vi "1125_group_6_project.vi"() -> ()   [LabVIEW 2016]
uses:
  <vilib>/DAQmx/write.llb/DAQmx Write (Digital Bool 1Line 1Point).vi
  <vilib>/DAQmx/create/channels.llb/DAQmx Create Channel (DO-Digital Output).vi
  <vilib>/DAQmx/miscellaneous.llb/DAQmx Fill In Error Info.vi
panel:
  in  "Pause":bool
  out "metal_flag":bool
  out "Efficiency":dbl
  out "Total Widgets":dbl
  out "plastic_flag":bool
  out "Widgets Failed":dbl
  out "Widgets Assembled":dbl
  out "Debug Counter":dbl
  out "elements 2":bool[](array[boolean])
  out "Hopper count":dbl
  out "latch for top thing":bool
  out "x > y?":bool
  out "reject/dont":bool
  out "elements":bool[](array[boolean])
  out "latch":bool
  out "laser near rejecter":bool
  out "laser latch":bool
  out "reject_laser":bool
  out "assm_check":bool
  out "bott_laser":bool
  out "bott_ind":bool
  out "bottom sensor":bool
  in  "Reset":bool
  out "ICT_stop":bool
  out "ICT_start":bool
  in  "stop":bool
  out "top_opt":bool
  out "top_ind":bool
  # "Normally On"
  # "Normally On"
  # "Normally On"
  # "Normally On"
  # "For backend data logging, ignore"
  # "Ignore, for debugging"
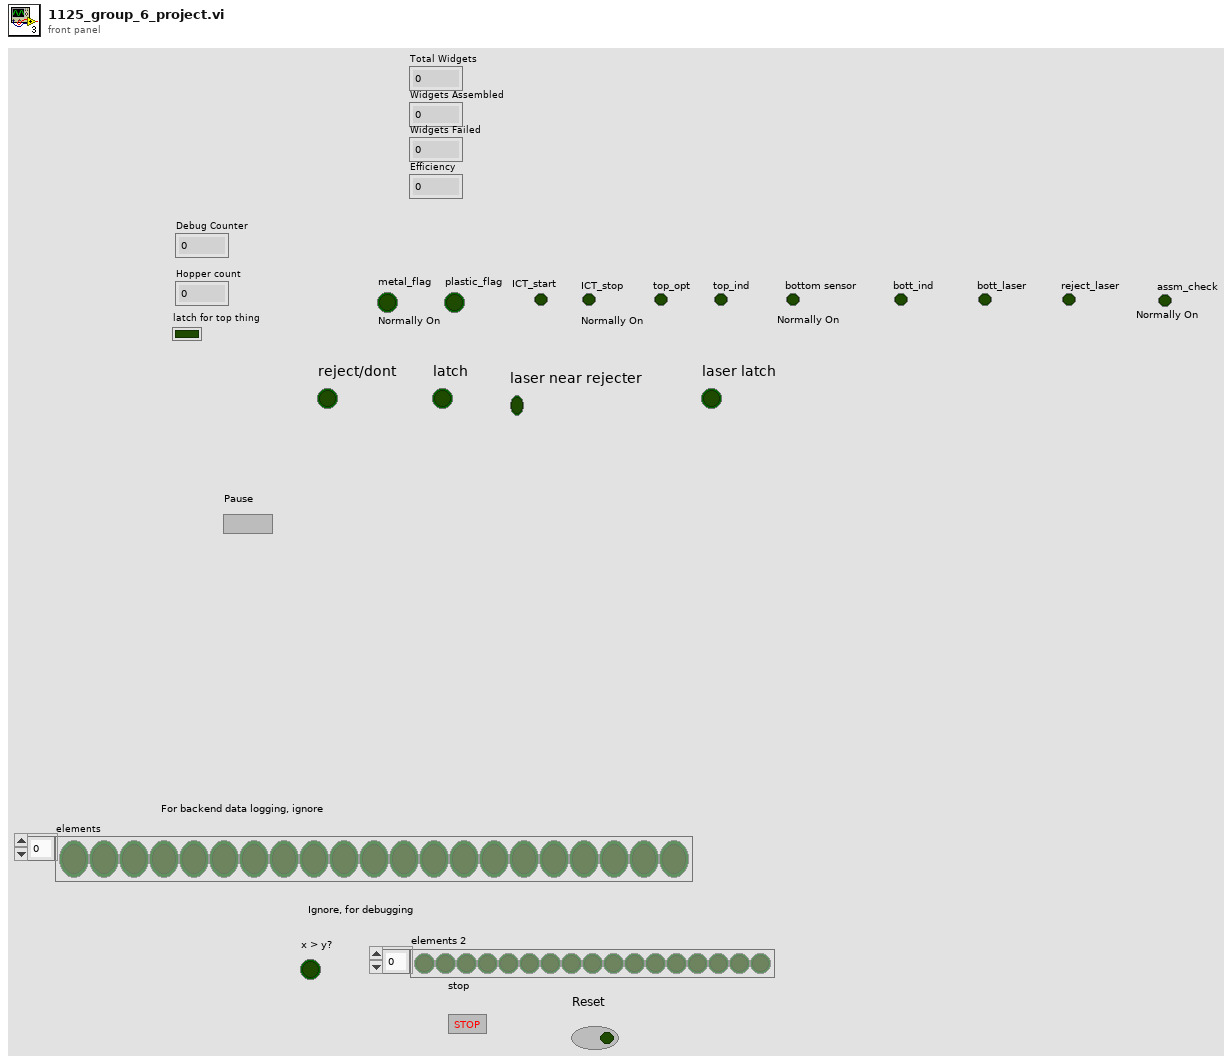
[diagram p1: front panel]
types:
  T1 = enum16{"open", "replace", "create", "open or create", "replace or create", "replace or create with confirmation"}
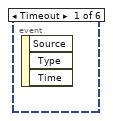
[diagram p4: hidden frame]
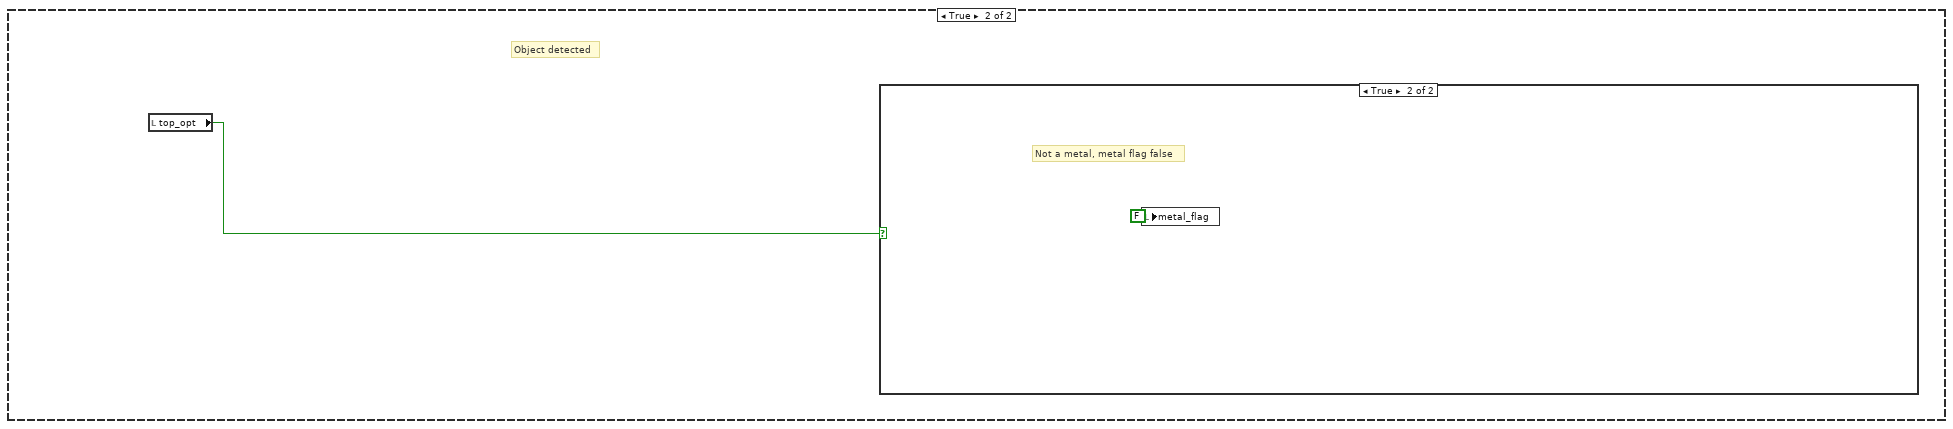
[diagram p8: hidden frame]
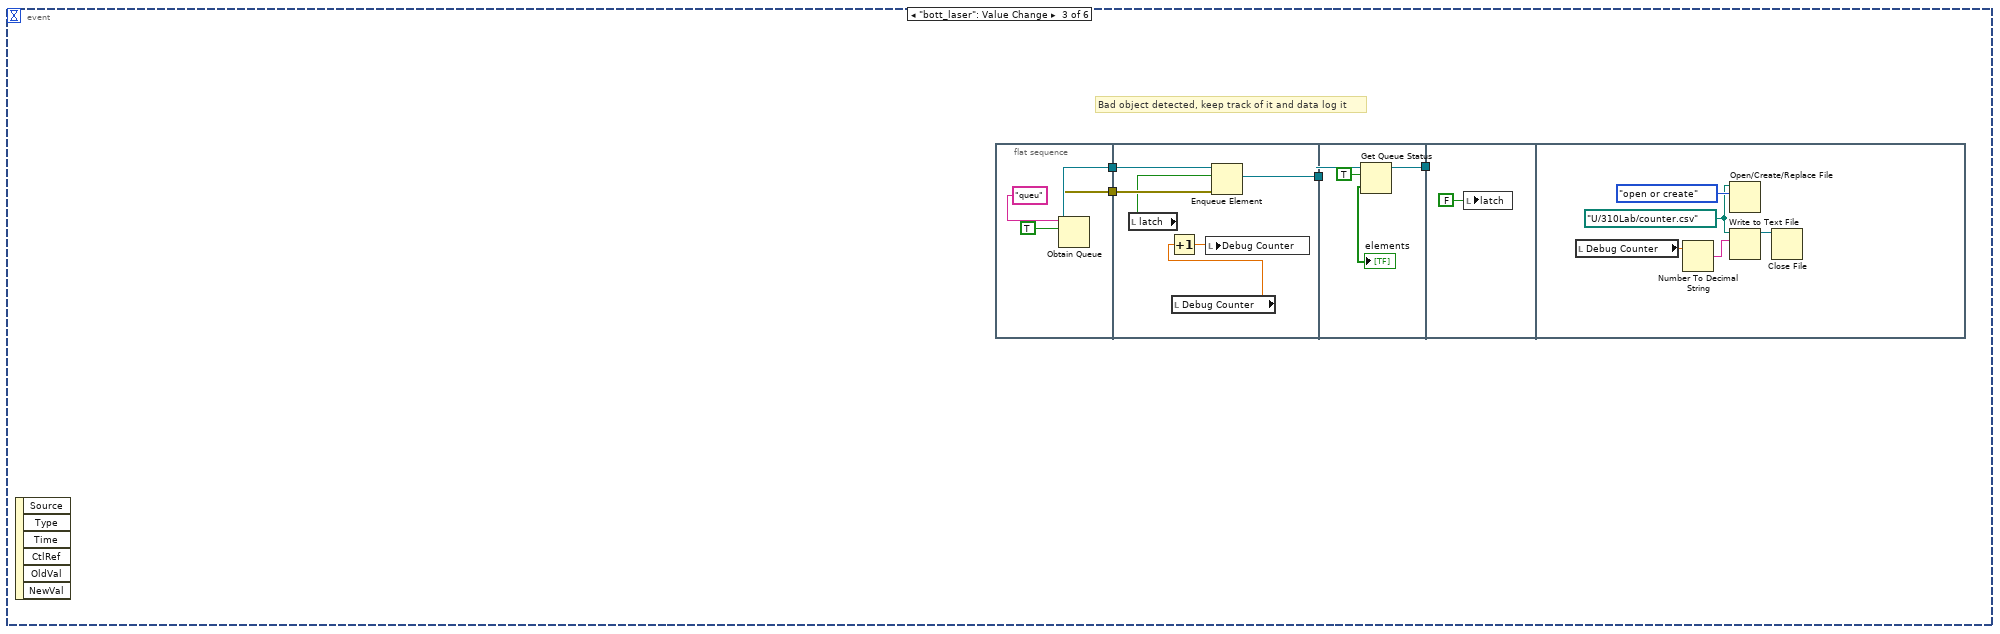
[diagram p10: hidden frame]
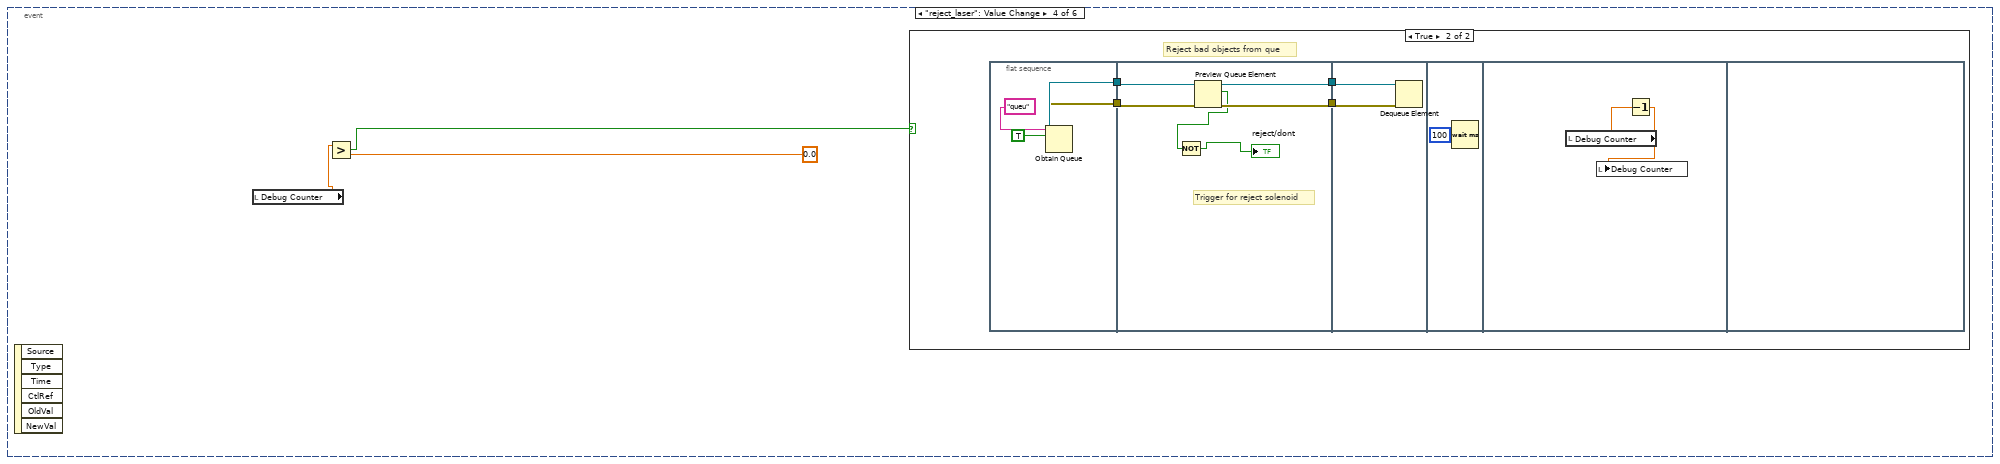
[diagram p11: hidden frame]
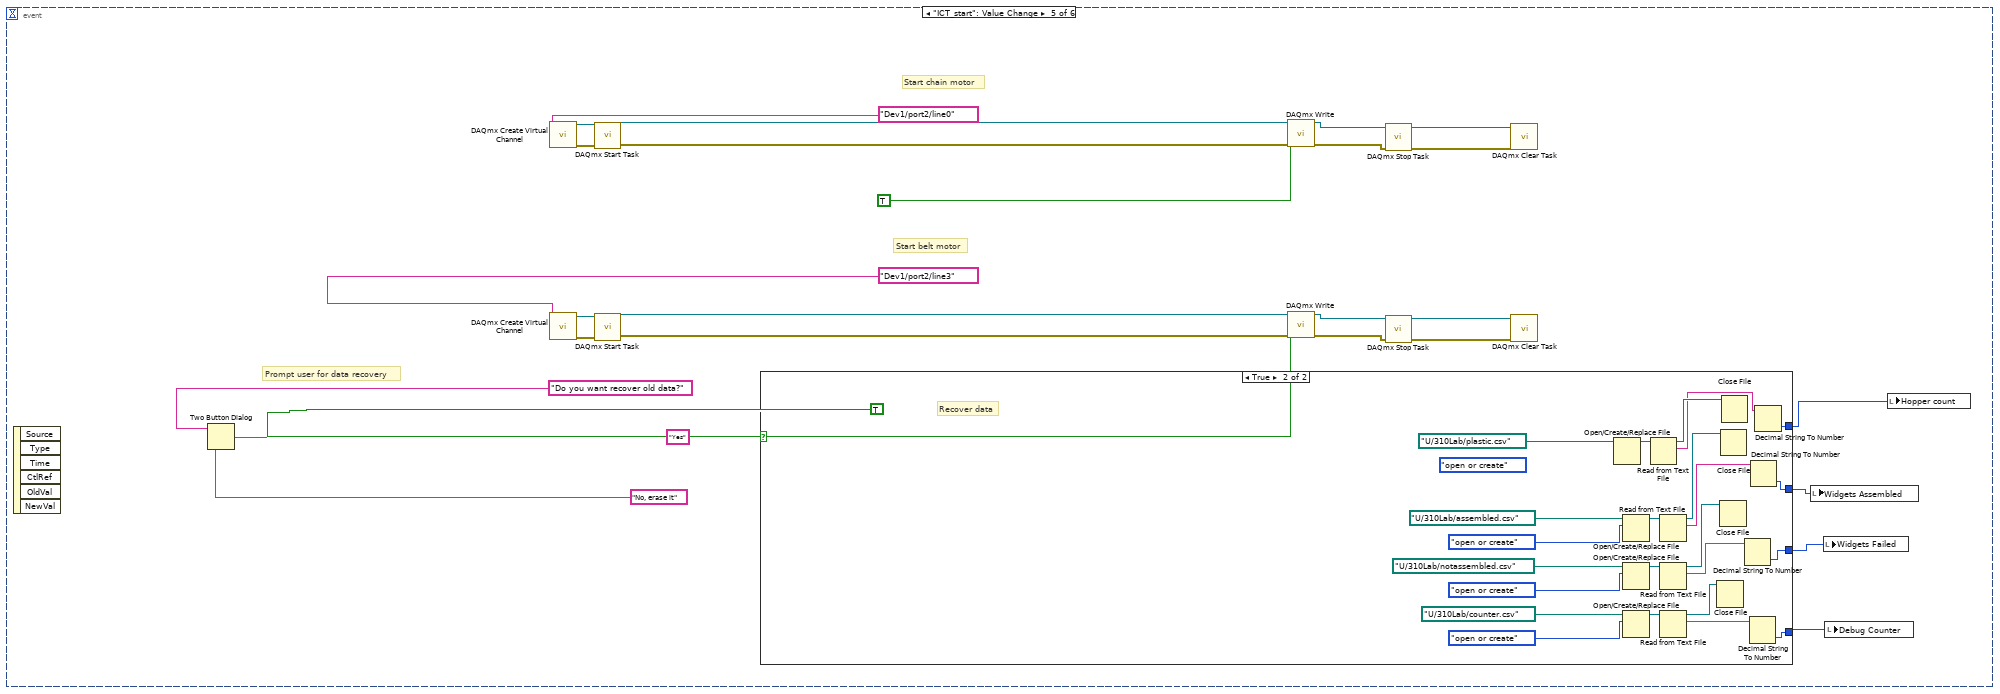
[diagram p13: hidden frame]
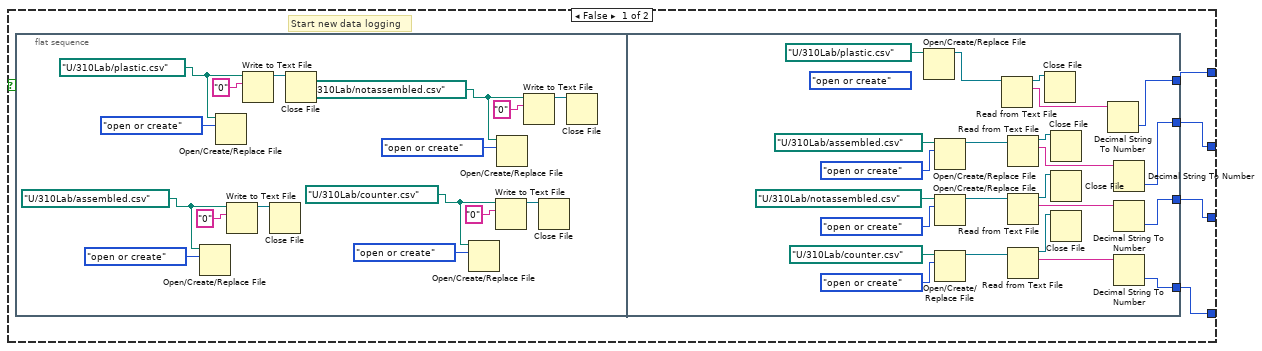
[diagram p14: hidden frame]
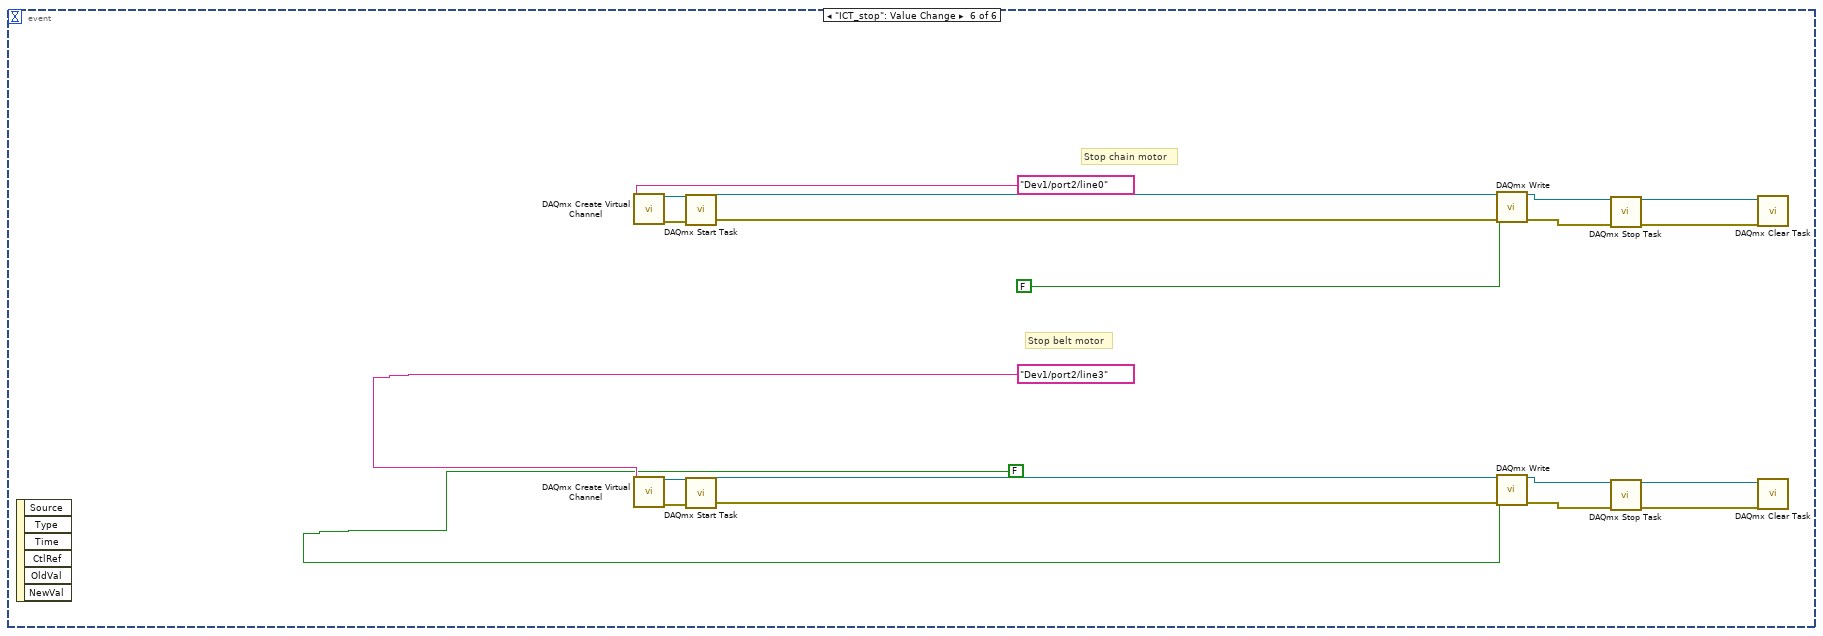
[diagram p15: hidden frame]
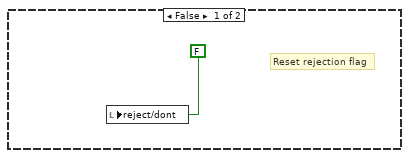
[diagram p19: hidden frame]
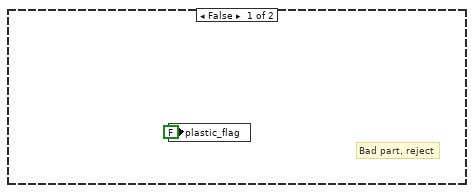
[diagram p20: hidden frame]
diagram:
  n1 = while {
    shift-right: [w60] -> _
    shift-left: _ -> [w61]
    shift-right: [w55] -> _
    shift-left: _ -> [w53]
    shift-right: [w51] -> _
    shift-left: _ -> [w50]
    shift-right: [w46] -> _
    shift-left: _ -> [w45]
    shift-right: [w39] -> _
    shift-left: _ -> [w36]
    shift-right: [w37] -> _
    shift-left: _ -> [w30]
    shift-right: [w38] -> _
    shift-left: _ -> [w28]
    shift-right: [w26] -> _
    shift-left: _ -> [w25]
    shift-right: [w21] -> _
    shift-left: _ -> [w20]
    shift-right: [w13] -> _
    shift-left: _ -> [w12]
    stop <- "stop" stop-if-true
    # "Bottom thing read vi"
    # "Bottom solenoid VI"
    # "Bottom metal sensor VI"
    # "Assembly check read VI"
    # "Dropper read VI"
    # "Stop button VI"
    # "Start button VI"
    # "Final Check"
    # "Shift registers to keep dynamic variables alive"
    # "Variables declaration"
    # "Reset all values stored (debugging purposes)"
    # "Ignore, for Debugging"
    # "Flag that metal is on chain"
    # "Read top_opt sensorr VI"
    # "Read top induct_sensor VI"
    # "Store top_opt status with shift register"
    # "Store top_ind status with shift register"
    # "Efficiency Calculation"
    n2 = local read "Widgets Assembled"() -> (w6:dbl)
    n3 = local read "Widgets Failed"() -> (w9:dbl)
    n4 = flat-sequence {
      frame #0 {
        n5 = event shown="[1] \"top_opt\": Value Change" {
          selector: _ -> [_ _ _ _ _ _]
          dyn-events: _ -> [_ _ _ _ _ _]
          timeout: 10 -> [_ _ _ _ _ _]
          event Timeout {
            n6 = event-data() -> ()  [unwired: 1 in, 3 out]
          }
          event "top_opt": Value Change {
            n7 = event-data() -> ()  [unwired: 1 in, 6 out]
            n8 = local read "top_ind"() -> (w73:bool)
            n9 = case shown="False" w73 {
              frame False {
                # "No object at top"
                n10 = local read "metal_flag"() -> (w74:bool)
                n11 = case shown="True" w74 {
                  frame False {
                  }
                  frame True {
                    # "Metal en route"
                    n12 = local read "top_opt"() -> (w75:bool)
                    n13 = case shown="True" w75 {
                      frame False {
                      }
                      frame True {
                        # "Check hopper"
                        # "Plastic ready"
                        n14 = local read "Hopper count"() -> (w77:dbl)
                        n15 = Less?(x=w77, y=5.0) -> (x < y?=w76:bool)
                        n16 = case shown="True" w76 {
                          frame False {
                          }
                          frame True {
                            # "Hopper not full, trigger sequence to add plastic to hopper"
                            n17 = flat-sequence {
                              frame #0 {
                                # "Stop belt motor"
                                n18 = call "1125_digital_write.vi"("lines"=tag "Dev1/port2/line3", "top ac"=FALSE ("top ac 2")) -> ()  [unwired: 10 in]
                              }
                              frame #1 {
                                # "Stop chain motor"
                                n19 = call "1125_digital_write.vi"("lines"=tag "Dev1/port2/line0", "top ac"=FALSE ("top ac 2")) -> ()  [unwired: 10 in]
                              }
                              frame #2 {
                                # "Enable sort solenoid"
                                n20 = call "1125_digital_write.vi"("lines"=tag "Dev1/port2/line1", "top ac"=TRUE ("top ac 2")) -> ()  [unwired: 10 in]
                              }
                              frame #3 {
                                n21 = Wait (ms)(milliseconds to wait=u32 500) -> ()  [unwired: 1 out]
                              }
                              frame #4 {
                                n22 = Wait (ms)(milliseconds to wait=u32 300) -> ()  [unwired: 1 out]
                              }
                              frame #5 {
                                # "Disable sort solenoid"
                                n23 = call "1125_digital_write.vi"("lines"=tag "Dev1/port2/line1", "top ac"=FALSE ("top ac 2")) -> ()  [unwired: 10 in]
                              }
                              frame #6 {
                                # "Add to hopper count"
                                n24 = local read "Hopper count"() -> (w90:dbl)
                                n25 = Add(x=w90, y=1.0) -> (x+y=w91:dbl)
                                n26 = local write "Hopper count"(w91) -> ()
                              }
                              frame #7 {
                                w95 = path "U:/310Lab/plastic.csv" ("file path (use dialog)")
                                # "Log hopper status"
                                n27 = local read "Hopper count"() -> (w94:dbl)
                                n28 = Number To Decimal String(number=w94) -> (decimal integer string=w93:string)  [unwired: 1 in]
                                n29 = Open/Create/Replace File(file path (use dialog)=w95, operation (0:open)=T1."open or create") -> ()  [unwired: 4 in, 3 out]
                                n30 = Write to Text File(file (use dialog)=w95, text=w93) -> (refnum out=w92:refnum<file>)  [unwired: 2 in, 2 out]
                                n31 = Close File(refnum=w92) -> ()  [unwired: 1 in, 2 out]
                              }
                              frame #8 {
                                # "Start belt motor"
                                n32 = call "1125_digital_write.vi"("lines"=tag "Dev1/port2/line0", "top ac"=TRUE ("top ac 2")) -> ()  [unwired: 10 in]
                              }
                              frame #9 {
                                # "Start chain motor"
                                n33 = call "1125_digital_write.vi"("lines"=tag "Dev1/port2/line3", "top ac"=TRUE ("top ac 2")) -> ()  [unwired: 10 in]
                              }
                            }
                          }
                        }
                      }
                    }
                  }
                }
              }
              frame True {
                # "Object detected"
                n34 = local read "top_opt"() -> (w101:bool)
                n35 = case shown="True" w101 {
                  frame False {
                  }
                  frame True {
                    # "Not a metal, metal flag false"
                    n36 = local write "metal_flag"(FALSE ("flag 2")) -> ()
                  }
                }
              }
            }
          }
          event "bott_laser": Value Change {
            # "Bad object detected, keep track of it and data log it"
            n37 = event-data() -> ()  [unwired: 1 in, 6 out]
            n38 = flat-sequence {
              tunnel: [w108] -> w106
              tunnel: [w107] -> w105
              tunnel: [w113] -> w104
              tunnel: w106 -> [w116]
              tunnel: w105 -> [w115]
              tunnel: w104 -> [w118]
              tunnel: [w117] -> w103
              tunnel: w103 -> [_]
              frame #0 {
                n39 = Obtain Queue(name (unnamed)="queu", element data type=TRUE ("latch bot")) -> (queue out=w108:refnum<queue>, error out=w107:errorcluster)  [unwired: 3 in, 1 out]
              }
              frame #1 {
                n40 = local read "latch"() -> (w114:bool)
                n41 = local read "Debug Counter"() -> (w111:dbl)
                n42 = Increment(x=w111) -> (x+1=w112:dbl)
                n43 = local write "Debug Counter"(w112) -> ()
                n44 = Enqueue Element(queue=w116, element=w114, error in (no error)=w115) -> (queue out=w113:refnum<queue>)  [unwired: 1 in, 2 out]
              }
              frame #2 {
                n45 = Get Queue Status(queue=w118, return elements? (F)=TRUE) -> (queue out=w117:refnum<queue>, elements=→"elements":bool[])  [unwired: 1 in, 6 out]
              }
              frame #3 {
                n46 = local write "latch"(FALSE ("latch bot")) -> ()
              }
              frame #4 {
                w125 = path "U:/310Lab/counter.csv" ("file path (use dialog)")
                n47 = local read "Debug Counter"() -> (w124:dbl)
                n48 = Number To Decimal String(number=w124) -> (decimal integer string=w123:string)  [unwired: 1 in]
                n49 = Open/Create/Replace File(file path (use dialog)=w125, operation (0:open)=T1."open or create") -> ()  [unwired: 4 in, 3 out]
                n50 = Write to Text File(file (use dialog)=w125, text=w123) -> (refnum out=w122:refnum<file>)  [unwired: 2 in, 2 out]
                n51 = Close File(refnum=w122) -> ()  [unwired: 1 in, 2 out]
              }
            }
          }
          event "reject_laser": Value Change {
            n52 = event-data() -> ()  [unwired: 1 in, 6 out]
            n53 = local read "Debug Counter"() -> (w129:dbl)
            n54 = Greater?(x=w129, y=0.0) -> (0:w127:bool)
            n55 = case shown="True" w127 {
              frame False {
                # "No bad objects in que"
              }
              frame True {
                # "Reject bad objects from que"
                n56 = flat-sequence {
                  tunnel: [w135] -> w132
                  tunnel: [w134] -> w133
                  tunnel: w133 -> [w139]
                  tunnel: [w141] -> w130
                  tunnel: w132 -> [w143]
                  tunnel: [w142] -> w131
                  tunnel: w131 -> [w145]
                  tunnel: w130 -> [w144]
                  frame #0 {
                    n57 = Obtain Queue(name (unnamed)="queu", element data type=TRUE ("latch bot")) -> (queue out=w135:refnum<queue>, error out=w134:errorcluster)  [unwired: 3 in, 1 out]
                  }
                  frame #1 {
                    # "Trigger for reject solenoid"
                    n58 = Preview Queue Element(queue=w143, error in (no error)=w139) -> (queue out=w142:refnum<queue>, element=w140:bool, error out=w141:errorcluster)  [unwired: 1 in, 1 out]
                    n59 = Not(x=w140) -> (.not. x?=→"reject/dont":bool)
                  }
                  frame #2 {
                    n60 = Dequeue Element(queue=w145, error in (no error)=w144) -> ()  [unwired: 1 in, 4 out]
                  }
                  frame #3 {
                    n61 = Wait (ms)(milliseconds to wait=u32 100) -> ()  [unwired: 1 out]
                  }
                  frame #4 {
                    n62 = local read "Debug Counter"() -> (w148:dbl)
                    n63 = Decrement(x=w148) -> (x-1=w147:dbl)
                    n64 = local write "Debug Counter"(w147) -> ()
                  }
                  frame #5 {
                  }
                }
              }
            }
          }
          event "ICT_start": Value Change {
            # "Prompt user for data recovery"
            # "Start belt motor"
            # "Start chain motor"
            n65 = event-data() -> ()  [unwired: 1 in, 6 out]
            n66 = Two Button Dialog(message="Do you want recover old data?", 1:"No, erase it" ("F button name (\"Cancel\")"), 2:"Yes" ("T button name (\"OK\")")) -> (T button?=w153:bool)
            n67 = call-poly <vilib>:"DAQmx Create Virtual Channel.vi"("lines"=tag "Dev1/port2/line0") -> ("task out"=w175:refnum<k21>, "error out"=w174:errorcluster)  [unwired: 13 in]
            n68 = call-poly <vilib>:"DAQmx Create Virtual Channel.vi"("lines"=tag "Dev1/port2/line3") -> ("task out"=w160:refnum<k21>, "error out"=w161:errorcluster)  [unwired: 13 in]
            n69 = call <vilib>:"DAQmx Start Task.vi"("task/channels in"=w175, "error in"=w174) -> ("task out"=w171:refnum<k21>, "error out"=w168:errorcluster)  [unwired: 12 in]
            n70 = call <vilib>:"DAQmx Start Task.vi"("task/channels in"=w160, "error in"=w161) -> ("task out"=w164:refnum<k21>, "error out"=w167:errorcluster)  [unwired: 12 in]
            n71 = case shown="True" w153 {
              tunnel: [w180 w230] -> w149
              tunnel: [w178 w229] -> w151
              tunnel: [w179 w228] -> w150
              tunnel: [w177 w220] -> w152
              frame False {
                # "Start new data logging"
                n72 = flat-sequence {
                  tunnel: [w217] -> w180
                  tunnel: [w214] -> w179
                  tunnel: [w211] -> w178
                  tunnel: [w197] -> w177
                  frame #0 {
                    w184 = path "U:/310Lab/notassembled.csv" ("file path (use dialog)")
                    w185 = path "U:/310Lab/counter.csv" ("file path (use dialog)")
                    w192 = path "U:/310Lab/assembled.csv" ("file path (use dialog)")
                    w193 = path "U:/310Lab/plastic.csv" ("file path (use dialog)")
                    n73 = Open/Create/Replace File(file path (use dialog)=w192, operation (0:open)=T1."open or create") -> ()  [unwired: 4 in, 3 out]
                    n74 = Open/Create/Replace File(file path (use dialog)=w193, operation (0:open)=T1."open or create") -> ()  [unwired: 4 in, 3 out]
                    n75 = Write to Text File(file (use dialog)=w192, text="0") -> (refnum out=w190:refnum<file>)  [unwired: 2 in, 2 out]
                    n76 = Write to Text File(file (use dialog)=w193, text="0") -> (refnum out=w195:refnum<file>)  [unwired: 2 in, 2 out]
                    n77 = Close File(refnum=w190) -> ()  [unwired: 1 in, 2 out]
                    n78 = Close File(refnum=w195) -> ()  [unwired: 1 in, 2 out]
                    n79 = Open/Create/Replace File(file path (use dialog)=w185, operation (0:open)=T1."open or create") -> ()  [unwired: 4 in, 3 out]
                    n80 = Write to Text File(file (use dialog)=w185, text="0") -> (refnum out=w187:refnum<file>)  [unwired: 2 in, 2 out]
                    n81 = Open/Create/Replace File(file path (use dialog)=w184, operation (0:open)=T1."open or create") -> ()  [unwired: 4 in, 3 out]
                    n82 = Write to Text File(file (use dialog)=w184, text="0") -> (refnum out=w182:refnum<file>)  [unwired: 2 in, 2 out]
                    n83 = Close File(refnum=w187) -> ()  [unwired: 1 in, 2 out]
                    n84 = Close File(refnum=w182) -> ()  [unwired: 1 in, 2 out]
                  }
                  frame #1 {
                    (unwired) T1."open or create" ("operation (0:open)")
                    n85 = Open/Create/Replace File(file path (use dialog)=path "U:/310Lab/plastic.csv") -> (refnum out=w198:refnum<file>)  [unwired: 5 in, 2 out]
                    n86 = Open/Create/Replace File(file path (use dialog)=path "U:/310Lab/assembled.csv", operation (0:open)=T1."open or create") -> (refnum out=w201:refnum<file>)  [unwired: 4 in, 2 out]
                    n87 = Open/Create/Replace File(file path (use dialog)=path "U:/310Lab/notassembled.csv", operation (0:open)=T1."open or create") -> (refnum out=w202:refnum<file>)  [unwired: 4 in, 2 out]
                    n88 = Open/Create/Replace File(file path (use dialog)=path "U:/310Lab/counter.csv", operation (0:open)=T1."open or create") -> (refnum out=w203:refnum<file>)  [unwired: 4 in, 2 out]
                    n89 = Read from Text File(file (use dialog)=w198) -> (refnum out=w199:refnum<file>, text=w200:string)  [unwired: 3 in, 2 out]
                    n90 = Read from Text File(file (use dialog)=w201) -> (refnum out=w213:refnum<file>, text=w212:string)  [unwired: 3 in, 2 out]
                    n91 = Read from Text File(file (use dialog)=w202) -> (refnum out=w215:refnum<file>, text=w216:string)  [unwired: 3 in, 2 out]
                    n92 = Read from Text File(file (use dialog)=w203) -> (refnum out=w219:refnum<file>, text=w218:string)  [unwired: 3 in, 2 out]
                    n93 = Close File(refnum=w199) -> ()  [unwired: 1 in, 2 out]
                    n94 = Close File(refnum=w213) -> ()  [unwired: 1 in, 2 out]
                    n95 = Close File(refnum=w215) -> ()  [unwired: 1 in, 2 out]
                    n96 = Close File(refnum=w219) -> ()  [unwired: 1 in, 2 out]
                    n97 = Decimal String To Number(string=w200) -> (number=w197:i32)  [unwired: 2 in, 1 out]
                    n98 = Decimal String To Number(string=w212) -> (number=w211:i32)  [unwired: 2 in, 1 out]
                    n99 = Decimal String To Number(string=w216) -> (number=w214:i32)  [unwired: 2 in, 1 out]
                    n100 = Decimal String To Number(string=w218) -> (number=w217:i32)  [unwired: 2 in, 1 out]
                  }
                }
              }
              frame True {
                (unwired) T1."open or create" ("operation (0:open)")
                # "Recover data"
                n101 = Open/Create/Replace File(file path (use dialog)=path "U:/310Lab/plastic.csv") -> (refnum out=w224:refnum<file>)  [unwired: 5 in, 2 out]
                n102 = Open/Create/Replace File(file path (use dialog)=path "U:/310Lab/assembled.csv", operation (0:open)=T1."open or create") -> (refnum out=w237:refnum<file>)  [unwired: 4 in, 2 out]
                n103 = Open/Create/Replace File(file path (use dialog)=path "U:/310Lab/notassembled.csv", operation (0:open)=T1."open or create") -> (refnum out=w240:refnum<file>)  [unwired: 4 in, 2 out]
                n104 = Open/Create/Replace File(file path (use dialog)=path "U:/310Lab/counter.csv", operation (0:open)=T1."open or create") -> (refnum out=w232:refnum<file>)  [unwired: 4 in, 2 out]
                n105 = Read from Text File(file (use dialog)=w224) -> (refnum out=w222:refnum<file>, text=w221:string)  [unwired: 3 in, 2 out]
                n106 = Read from Text File(file (use dialog)=w237) -> (refnum out=w235:refnum<file>, text=w236:string)  [unwired: 3 in, 2 out]
                n107 = Read from Text File(file (use dialog)=w240) -> (refnum out=w242:refnum<file>, text=w241:string)  [unwired: 3 in, 2 out]
                n108 = Read from Text File(file (use dialog)=w232) -> (refnum out=w234:refnum<file>, text=w233:string)  [unwired: 3 in, 2 out]
                n109 = Close File(refnum=w234) -> ()  [unwired: 1 in, 2 out]
                n110 = Close File(refnum=w242) -> ()  [unwired: 1 in, 2 out]
                n111 = Close File(refnum=w235) -> ()  [unwired: 1 in, 2 out]
                n112 = Close File(refnum=w222) -> ()  [unwired: 1 in, 2 out]
                n113 = Decimal String To Number(string=w241) -> (number=w228:i32)  [unwired: 2 in, 1 out]
                n114 = Decimal String To Number(string=w233) -> (number=w230:i32)  [unwired: 2 in, 1 out]
                n115 = Decimal String To Number(string=w236) -> (number=w229:i32)  [unwired: 2 in, 1 out]
                n116 = Decimal String To Number(string=w221) -> (number=w220:i32)  [unwired: 2 in, 1 out]
              }
            }
            n117 = call-poly <vilib>:"DAQmx Write.vi"("task/channels in"=w171, "data"=TRUE, "error in"=w168) -> ("task out"=w170:refnum<k21>, "error out"=w169:errorcluster)  [unwired: 10 in, 1 out]
            n118 = call-poly <vilib>:"DAQmx Write.vi"("task/channels in"=w164, "data"=TRUE, "error in"=w167) -> ("task out"=w165:refnum<k21>, "error out"=w166:errorcluster)  [unwired: 10 in, 1 out]
            n119 = call <vilib>:"DAQmx Stop Task.vi"("task/channels in"=w170, "error in"=w169) -> ("task out"=w173:refnum<k21>, "error out"=w172:errorcluster)  [unwired: 12 in]
            n120 = call <vilib>:"DAQmx Stop Task.vi"("task/channels in"=w165, "error in"=w166) -> ("task out"=w162:refnum<k21>, "error out"=w163:errorcluster)  [unwired: 12 in]
            n121 = call <vilib>:"DAQmx Clear Task.vi"("task in"=w173, "error in"=w172) -> ()  [unwired: 13 in, 1 out]
            n122 = call <vilib>:"DAQmx Clear Task.vi"("task in"=w162, "error in"=w163) -> ()  [unwired: 13 in, 1 out]
            n123 = local write "Widgets Assembled"(w151) -> ()
            n124 = local write "Widgets Failed"(w150) -> ()
            n125 = local write "Debug Counter"(w149) -> ()
            n126 = local write "Hopper count"(w152) -> ()
          }
          event "ICT_stop": Value Change {
            # "Stop belt motor"
            # "Stop chain motor"
            n127 = event-data() -> ()  [unwired: 1 in, 6 out]
            n128 = call-poly <vilib>:"DAQmx Create Virtual Channel.vi"("lines"=tag "Dev1/port2/line0") -> ("task out"=w261:refnum<k21>, "error out"=w260:errorcluster)  [unwired: 13 in]
            n129 = call-poly <vilib>:"DAQmx Create Virtual Channel.vi"("lines"=tag "Dev1/port2/line3") -> ("task out"=w246:refnum<k21>, "error out"=w247:errorcluster)  [unwired: 13 in]
            n130 = call <vilib>:"DAQmx Start Task.vi"("task/channels in"=w261, "error in"=w260) -> ("task out"=w257:refnum<k21>, "error out"=w254:errorcluster)  [unwired: 12 in]
            n131 = call <vilib>:"DAQmx Start Task.vi"("task/channels in"=w246, "error in"=w247) -> ("task out"=w250:refnum<k21>, "error out"=w253:errorcluster)  [unwired: 12 in]
            n132 = call-poly <vilib>:"DAQmx Write.vi"("task/channels in"=w257, "data"=FALSE, "error in"=w254) -> ("task out"=w256:refnum<k21>, "error out"=w255:errorcluster)  [unwired: 10 in, 1 out]
            n133 = call-poly <vilib>:"DAQmx Write.vi"("task/channels in"=w250, "data"=FALSE, "error in"=w253) -> ("task out"=w251:refnum<k21>, "error out"=w252:errorcluster)  [unwired: 10 in, 1 out]
            n134 = call <vilib>:"DAQmx Stop Task.vi"("task/channels in"=w256, "error in"=w255) -> ("task out"=w259:refnum<k21>, "error out"=w258:errorcluster)  [unwired: 12 in]
            n135 = call <vilib>:"DAQmx Stop Task.vi"("task/channels in"=w251, "error in"=w252) -> ("task out"=w248:refnum<k21>, "error out"=w249:errorcluster)  [unwired: 12 in]
            n136 = call <vilib>:"DAQmx Clear Task.vi"("task in"=w259, "error in"=w258) -> ()  [unwired: 13 in, 1 out]
            n137 = call <vilib>:"DAQmx Clear Task.vi"("task in"=w248, "error in"=w249) -> ()  [unwired: 13 in, 1 out]
          }
        }
      }
      frame #1 {
        n138 = local read "bottom sensor"() -> (w263:bool)
        n139 = case shown="False" w263 {
          frame False {
            # "Note that this is an inductive sensor"
            # "Check that plastic in hopper"
            # "Normally on, so trigger this sequence when off (object in front of bottom sensor)"
            n140 = local read "Hopper count"() -> (w266:dbl)
            n141 = Greater?(x=w266, y=0.0) -> (0:w264:bool)
            n142 = case shown="True" w264 {
              frame False {
                # "This too shall pass"
              }
              frame True {
                n143 = flat-sequence {
                  frame #0 {
                    # "Wait for metal to collect plastic\nand pass by"
                    n144 = Wait (ms)(milliseconds to wait=u32 400) -> ()  [unwired: 1 out]
                  }
                  frame #1 {
                    # "Stop belt motor"
                    n145 = call "1125_digital_write.vi"("lines"=tag "Dev1/port2/line3", "top ac"=FALSE ("top ac 2")) -> ()  [unwired: 10 in]
                  }
                  frame #2 {
                    # "Stop chain motor"
                    n146 = call "1125_digital_write.vi"("lines"=tag "Dev1/port2/line0", "top ac"=FALSE ("top ac 2")) -> ()  [unwired: 10 in]
                  }
                  frame #3 {
                    # "Trigger rotary to\nrelease plastic"
                    n147 = call "1125_rotary_write.vi"("Boolean"=TRUE) -> ()  [unwired: 11 in]
                  }
                  frame #4 {
                    n148 = Wait (ms)(milliseconds to wait=u32 400) -> ()  [unwired: 1 out]
                  }
                  frame #5 {
                    # "Disable rotary"
                    n149 = call "1125_rotary_write.vi"("Boolean"=FALSE) -> ()  [unwired: 11 in]
                  }
                  frame #6 {
                    # "Let pieces in hopper settle"
                    n150 = Wait (ms)(milliseconds to wait=u32 250) -> ()  [unwired: 1 out]
                  }
                  frame #7 {
                    # "Subtract from count"
                    n151 = local read "Hopper count"() -> (w277:dbl)
                    n152 = Subtract(x=w277, y=1.0) -> (x-y=w278:dbl)
                    n153 = local write "Hopper count"(w278) -> ()
                  }
                  frame #8 {
                    # "Enable chain motor"
                    n154 = call "1125_digital_write.vi"("lines"=tag "Dev1/port2/line0", "top ac"=TRUE ("top ac 2")) -> ()  [unwired: 10 in]
                  }
                  frame #9 {
                    # "Enable belt motor"
                    n155 = call "1125_digital_write.vi"("lines"=tag "Dev1/port2/line3", "top ac"=TRUE ("top ac 2")) -> ()  [unwired: 10 in]
                  }
                }
              }
            }
          }
          frame True {
          }
        }
      }
    }
    n156 = local read "top_opt"() -> (w58:bool)
    n157 = local read "assm_check"() -> (w33:bool)
    n158 = local read "ICT_start"() -> (w54:bool)
    n159 = local read "top_ind"() -> (w14:bool)
    n160 = local read "reject/dont"() -> (w19:bool)
    n161 = local read "assm_check"() -> (w16:bool)
    n162 = Greater?(x=w54, y=w53) -> (0:w56:bool)
    n163 = local read "bott_ind"() -> (w35:bool)
    n164 = local read "ICT_stop"() -> (w44:bool)
    n165 = local read "bott_laser"() -> (w32:bool)
    n166 = local read "bottom sensor"() -> (w43:bool)
    n167 = Less?(x=w32, y=w30) -> (x < y?=w31:bool)
    n168 = local read "reject_laser"() -> (w27:bool)
    n169 = Greater?(x=w58, y=w61) -> (0:w59:bool)
    n170 = Less?(x=w33, y=w28) -> (x < y?=w24:bool)
    n171 = local read "bott_ind"() -> (w22:bool)
    n172 = Greater?(x=w19, y=w20) -> (0:w18:bool)
    n173 = Greater?(x=w35, y=w36) -> (0:w34:bool)
    n174 = Greater?(x=w14, y=w12) -> (0:w15:bool)
    "x > y?" <- w15
    n175 = Greater?(x=w27, y=w25) -> (0:w23:bool)
    n176 = Add(x=w6, y=w9) -> (x+y=w8:dbl)
    n177 = local read "Total Widgets"() -> (w5:dbl)
    n178 = case shown="True" w18 {
      frame False {
        # "Reset rejection flag"
        n179 = local write "reject/dont"(FALSE) -> ()
      }
      frame True {
        n180 = flat-sequence {
          frame #0 {
            # "Trigger reject \nsolenoid"
            n181 = call "1125_reject_solenoid_write.vi"("Boolean"=TRUE) -> ()  [unwired: 11 in]
          }
          frame #1 {
            n182 = Wait (ms)(milliseconds to wait=u32 80) -> ()  [unwired: 1 out]
          }
          frame #2 {
            # "Disable\nreject\nsolenoid"
            n183 = call "1125_reject_solenoid_write.vi"("Boolean"=FALSE) -> ()  [unwired: 11 in]
          }
          frame #3 {
            # "Add to failed widgets"
            n184 = local read "Widgets Failed"() -> (w289:dbl)
            n185 = Increment(x=w289) -> (x+1=w288:dbl)
            n186 = local write "Widgets Failed"(w288) -> ()
          }
          frame #4 {
            w291 = path "U:/310Lab/notassembled.csv" ("file path (use dialog)")
            # "Data log failure in CSV"
            n187 = local read "Widgets Failed"() -> (w292:dbl)
            n188 = Number To Decimal String(number=w292) -> (decimal integer string=w293:string)  [unwired: 1 in]
            n189 = Open/Create/Replace File(file path (use dialog)=w291, operation (0:open)=T1."open or create") -> ()  [unwired: 4 in, 3 out]
            n190 = Write to Text File(file (use dialog)=w291, text=w293) -> (refnum out=w294:refnum<file>)  [unwired: 2 in, 2 out]
            n191 = Close File(refnum=w294) -> ()  [unwired: 1 in, 2 out]
          }
        }
      }
    }
    n192 = local write "Total Widgets"(w8) -> ()
    n193 = Divide(x=w6, y=w5) -> (x/y=→"Efficiency":dbl)
    n194 = case shown="True" w56 {
      frame False {
      }
      frame True {
        n195 = property on="ICT_start" class="Bool (strict)"("Val(Sgnl)"=TRUE) -> ()  [unwired: 2 in, 2 out]
      }
    }
    n196 = Not(x=w16) -> (.not. x?=w17:bool)
    n197 = Greater?(x=w44, y=w50) -> (0:w52:bool)
    n198 = case shown="True" w24 {
      frame False {
      }
      frame True {
        n199 = Wait (ms)(milliseconds to wait=u32 10) -> ()  [unwired: 1 out]
        n200 = property on="assm_check" class="Bool (strict)"("Val(Sgnl)"=TRUE) -> ()  [unwired: 2 in, 2 out]
      }
    }
    n201 = And(x=w22, y=w17) -> (x .and. y?=w10:bool)
    n202 = case shown="True" w15 {
      frame False {
      }
      frame True {
        n203 = property on="top_ind" class="Bool (strict)"("Val(Sgnl)"=TRUE ("Value (Signaling)")) -> ()  [unwired: 2 in, 2 out]
      }
    }
    n204 = case shown="True" w34 {
      frame False {
      }
      frame True {
        n205 = property on="bott_ind" class="Bool (strict)"("Val(Sgnl)"=TRUE) -> ()  [unwired: 2 in, 2 out]
      }
    }
    n206 = case shown="True" w59 {
      frame False {
      }
      frame True {
        n207 = property on="top_opt" class="Bool (strict)"("Val(Sgnl)"=TRUE) -> ()  [unwired: 2 in, 2 out]
      }
    }
    n208 = Greater?(x=w43, y=w45) -> (0:w48:bool)
    n209 = case shown="True" w31 {
      frame False {
        n210 = local write "laser latch"(FALSE ("lazer latch")) -> ()
      }
      frame True {
        n211 = property on="bott_laser" class="Bool (strict)"("Val(Sgnl)"=TRUE) -> ()  [unwired: 2 in, 2 out]
        n212 = local write "laser latch"(TRUE) -> ()
      }
    }
    n213 = case shown="True" w23 {
      frame False {
        n214 = local write "laser near rejecter"(FALSE ("lazer near kicker")) -> ()
      }
      frame True {
        n215 = property on="reject_laser" class="Bool (strict)"("Val(Sgnl)"=TRUE) -> ()  [unwired: 2 in, 2 out]
        n216 = local write "laser near rejecter"(TRUE ("lazer near kicker")) -> ()
      }
    }
    n217 = call "1125_dropper_read.vi"() -> ("data"=→"bottom sensor":bool)  [unwired: 11 in]
    n218 = case shown="True" w52 {
      frame False {
      }
      frame True {
        n219 = property on="ICT_stop" class="Bool (strict)"("Val(Sgnl)"=TRUE) -> ()  [unwired: 2 in, 2 out]
      }
    }
    n220 = call "1125_start_butt_read.vi"() -> ("data 2"=→"ICT_start":bool)  [unwired: 11 in]
    n221 = call "1125_top_thing_read.vi"() -> ("data"=→"top_opt":bool)  [unwired: 11 in]
    n222 = call "1125_top_metal_read.vi"() -> ("data"=→"top_ind":bool)  [unwired: 11 in]
    n223 = case shown="True" w10 {
      frame False {
        # "Bad part, reject"
        n224 = local write "plastic_flag"(FALSE ("flag")) -> ()
      }
      frame True {
        # "Final check good"
        n225 = local read "plastic_flag"() -> (w296:bool)
        n226 = case shown="False" w296 {
          frame False {
            # "Not plastic"
            n227 = flat-sequence {
              frame #0 {
                # "Add  to assembly count"
                n228 = local read "Widgets Assembled"() -> (w298:dbl)
                n229 = Increment(x=w298) -> (x+1=w299:dbl)
                n230 = local write "Widgets Assembled"(w299) -> ()
              }
              frame #1 {
                n231 = local write "plastic_flag"(TRUE ("flag")) -> ()
              }
              frame #2 {
                w304 = path "U:/310Lab/assembled.csv" ("file path (use dialog)")
                n232 = local read "Widgets Assembled"() -> (w303:dbl)
                n233 = Number To Decimal String(number=w303) -> (decimal integer string=w302:string)  [unwired: 1 in]
                n234 = Open/Create/Replace File(file path (use dialog)=w304, operation (0:open)=T1."open or create") -> ()  [unwired: 4 in, 3 out]
                n235 = Write to Text File(file (use dialog)=w304, text=w302) -> (refnum out=w301:refnum<file>)  [unwired: 2 in, 2 out]
                n236 = Close File(refnum=w301) -> ()  [unwired: 1 in, 2 out]
              }
            }
          }
          frame True {
            # "This is redundant, but helps if something gets messed\nup with the machine."
            # "Is plastic, proceed to reject"
            n237 = local write "plastic_flag"(TRUE ("flag")) -> ()
          }
        }
        n238 = local write "latch"(TRUE ("latch")) -> ()
      }
    }
    n239 = case shown="True" TRUE {
      frame False {
      }
      frame True {
        n240 = Obtain Queue(name (unnamed)="queu", element data type=TRUE ("latch bot")) -> (queue out=w69:refnum<queue>, error out=w67:errorcluster)  [unwired: 3 in, 1 out]
        n241 = Get Queue Status(queue=w69, return elements? (F)=TRUE, error in (no error)=w67) -> (elements=→"elements 2":bool[])  [unwired: 7 out]
      }
    }
    n242 = local read "top_opt"() -> (w4:bool)
    n243 = case shown="False" w4 {
      frame False {
        n244 = local write "metal_flag"(TRUE ("flag 2")) -> ()
      }
      frame True {
      }
    }
    n245 = case shown="True" w48 {
      frame False {
        n246 = property on="latch for top thing" class="Bool (strict)"("Val(Sgnl)"=FALSE ("Value (Signaling)")) -> ()  [unwired: 2 in, 2 out]
      }
      frame True {
        n247 = property on="latch for top thing" class="Bool (strict)"("Val(Sgnl)"=TRUE ("Value (Signaling)")) -> ()  [unwired: 2 in, 2 out]
        n248 = property on="bottom sensor" class="Bool (strict)"("Val(Sgnl)"=FALSE) -> ()  [unwired: 2 in, 2 out]
      }
    }
    n249 = call "1125_stop_butt_read.vi"() -> ("data"=w3:bool)  [unwired: 11 in]
    n250 = Exclusive Or(1:"Pause", 2:w3) -> (0:→"ICT_stop":bool)
    n251 = call "1125_bott_soln_read.vi"() -> ("data"=→"bott_laser":bool)  [unwired: 11 in]
    n252 = call "1125_bott_thing_read.vi"() -> ("data"=→"reject_laser":bool)  [unwired: 11 in]
    n253 = call "1125_bott_metal_read.vi"() -> ("data"=→"bott_ind":bool)  [unwired: 11 in]
    n254 = call "1125_assm_read.vi"() -> ("data"=→"assm_check":bool)  [unwired: 11 in]
    n255 = case shown="True" "Reset" {
      frame False {
      }
      frame True {
        n256 = local write "Widgets Assembled"(0.0 ("Plastic count")) -> ()
        n257 = local write "Debug Counter"(0.0 ("Plastic count")) -> ()
        n258 = local write "Hopper count"(0.0 ("Plastic count")) -> ()
        n259 = local write "Widgets Failed"(0.0 ("Plastic count")) -> ()
      }
    }
    n260 = local read "assm_check"() -> (w38:bool)
    n261 = local read "bott_ind"() -> (w39:bool)
    n262 = local read "bott_laser"() -> (w37:bool)
    n263 = local read "reject_laser"() -> (w26:bool)
    n264 = local read "ICT_start"() -> (w55:bool)
    n265 = local read "reject/dont"() -> (w21:bool)
    n266 = local read "bottom sensor"() -> (w46:bool)
    n267 = local read "top_ind"() -> (w13:bool)
    n268 = local read "top_opt"() -> (w60:bool)
    n269 = local read "ICT_stop"() -> (w51:bool)
  }
